vi "工具.vi"() -> ()   [LabVIEW 2011]
panel:
  in  "字符串":string="#0 write #A0 #00 K#00 Z#128@#0 read #A1 #00 #128@#1 write #A0 #00 K#00 Z#128@#1 read #A1 #00 #128$#0 write #A0 #7F V#0@#0 read #A1 #80 #128@#1 write #A0 #7F V#0@#1 read #A1 #80 #128$#0 write #A0 #80 K#01 Z#128@#0 write #A0 #7F V#01@#1 write #A0 #80 K#01 Z#128@#1 write #A0 #7F V#01$#0 write #A0 #7F V#1@#0 read #A1 #80 #128@#1 write #A0 #7F V#1@#1 read #A1 #80 #128$#0 write #A0 #80 K#02 Z#128@#0 write #A0 #7F V#02@#1 write #A0 #80 K#02 Z#128@#1 write #A0 #7F V#02$#0 write #A0 #7F V#2@#0 write #A0 #7B K#10 Z#004@#1 write #A0 #7F V#2@#1 write #A0 #7B K#10 Z#004$#0 write #A0 #7B K#10 Z#004@#0 read #A1 #80 #128@#1 write #A0 #7B K#10 Z#004@#1 read #A1 #80 #128$#0 write #A0 #80 K#03 Z#128@#0 write #A0 #7F V#03@#1 write #A0 #80 K#03 Z#128@#1 write #A0 #7F V#03$#0 write #A0 #7F V#3@#0 read #A1 #80 #128@#1 write #A0 #7F V#3@#1 read #A1 #80 #128$#0 write #A0 #80 K#04 Z#128@#0 write #A0 #7F V#00@#1 write #A0 #80 K#04 Z#128@#1 write #A0 #7F V#00$#0 write #A0 #7F V#0@#0 write #A0 #7B K#11 Z#004@#1 write #A0 #7F V#0@#1 write #A0 #7B K#11 Z#004$#0 write #A0 #7B K#11 Z#004@@#1 write #A0 #7B K#11 Z#004@$@@@$@@@$\r"
  out "电子表格字符串":string="#0 write #A0 #00 K#00 Z#128@#0 read #A1 #00 #128@#1 write #A0 #00 K#00 Z#128@#1 read #A1 #00 #128$#0 write #A0 #7F V#0@#0 read #A1 #80 #128@#1 write #A0 #7F V#0@#1 read #A1 #80 #128$#0 write #A0 #80 K#01 Z#128@#0 write #A0 #7F V#01@#1 write #A0 #80 K#01 Z#128@#1 write #A0 #7F V#01$#0 write #A0 #7F V#1@#0 read #A1 #80 #128@#1 write #A0 #7F V#1@#1 read #A1 #80 #128$#0 write #A0 #80 K#02 Z#128@#0 write #A0 #7F V#02@#1 write #A0 #80 K#02 Z#128@#1 write #A0 #7F V#02$#0 write #A0 #7F V#2@#0 write #A0 #7B K#10 Z#004@#1 write #A0 #7F V#2@#1 write #A0 #7B K#10 Z#004$#0 write #A0 #7B K#10 Z#004@#0 read #A1 #80 #128@#1 write #A0 #7B K#10 Z#004@#1 read #A1 #80 #128$#0 write #A0 #80 K#03 Z#128@#0 write #A0 #7F V#03@#1 write #A0 #80 K#03 Z#128@#1 write #A0 #7F V#03$#0 write #A0 #7F V#3@#0 read #A1 #80 #128@#1 write #A0 #7F V#3@#1 read #A1 #80 #128$#0 write #A0 #80 K#04 Z#128@#0 write #A0 #7F V#00@#1 write #A0 #80 K#04 Z#128@#1 write #A0 #7F V#00$#0 write #A0 #7F V#0@#0 write #A0 #7B K#11 Z#004@#1 write #A0 #7F V#0@#1 write #A0 #7B K#11 Z#004$#0 write #A0 #7B K#11 Z#004@@#1 write #A0 #7B K#11 Z#004@$@@@$@@@$@@@$"
  out "数组":string[][](array[string])=[["#0 write #A0 #00 K#00 Z#128", "#0 read #A1 #00 #128", "#1 write #A0 #00 K#00 Z#128", "#1 read #A1 #00 #128"], ["#0 write #A0 #7F V#0", "#0 read #A1 #80 #128", "#1 write #A0 #7F V#0", "#1 read #A1 #80 #128"], ["#0 write #A0 #80 K#01 Z#128", "#0 write #A0 #7F V#01", "#1 write #A0 #80 K#01 Z#128", "#1 write #A0 #7F V#01"], ["#0 write #A0 #7F V#1", "#0 read #A1 #80 #128", "#1 write #A0 #7F V#1", "#1 read #A1 #80 #128"], ["#0 write #A0 #80 K#02 Z#128", "#0 write #A0 #7F V#02", "#1 write #A0 #80 K#02 Z#128", "#1 write #A0 #7F V#02"], ["#0 write #A0 #7F V#2", "#0 write #A0 #7B K#10 Z#004", "#1 write #A0 #7F V#2", "#1 write #A0 #7B K#10 Z#004"], ["#0 write #A0 #7B K#10 Z#004", "#0 read #A1 #80 #128", "#1 write #A0 #7B K#10 Z#004", "#1 read #A1 #80 #128"], ["#0 write #A0 #80 K#03 Z#128", "#0 write #A0 #7F V#03", "#1 write #A0 #80 K#03 Z#128", "#1 write #A0 #7F V#03"], ["#0 write #A0 #7F V#3", "#0 read #A1 #80 #128", "#1 write #A0 #7F V#3", "#1 read #A1 #80 #128"], ["#0 write #A0 #80 K#04 Z#128", "#0 write #A0 #7F V#00", "#1 write #A0 #80 K#04 Z#128", "#1 write #A0 #7F V#00"], ["#0 write #A0 #7F V#0", "#0 write #A0 #7B K#11 Z#004", "#1 write #A0 #7F V#0", "#1 write #A0 #7B K#11 Z#004"], ["#0 write #A0 #7B K#11 Z#004", "", "#1 write #A0 #7B K#11 Z#004", ""], ["", "", "", ""], ["", "", "", ""], ["", "", "", ""]]
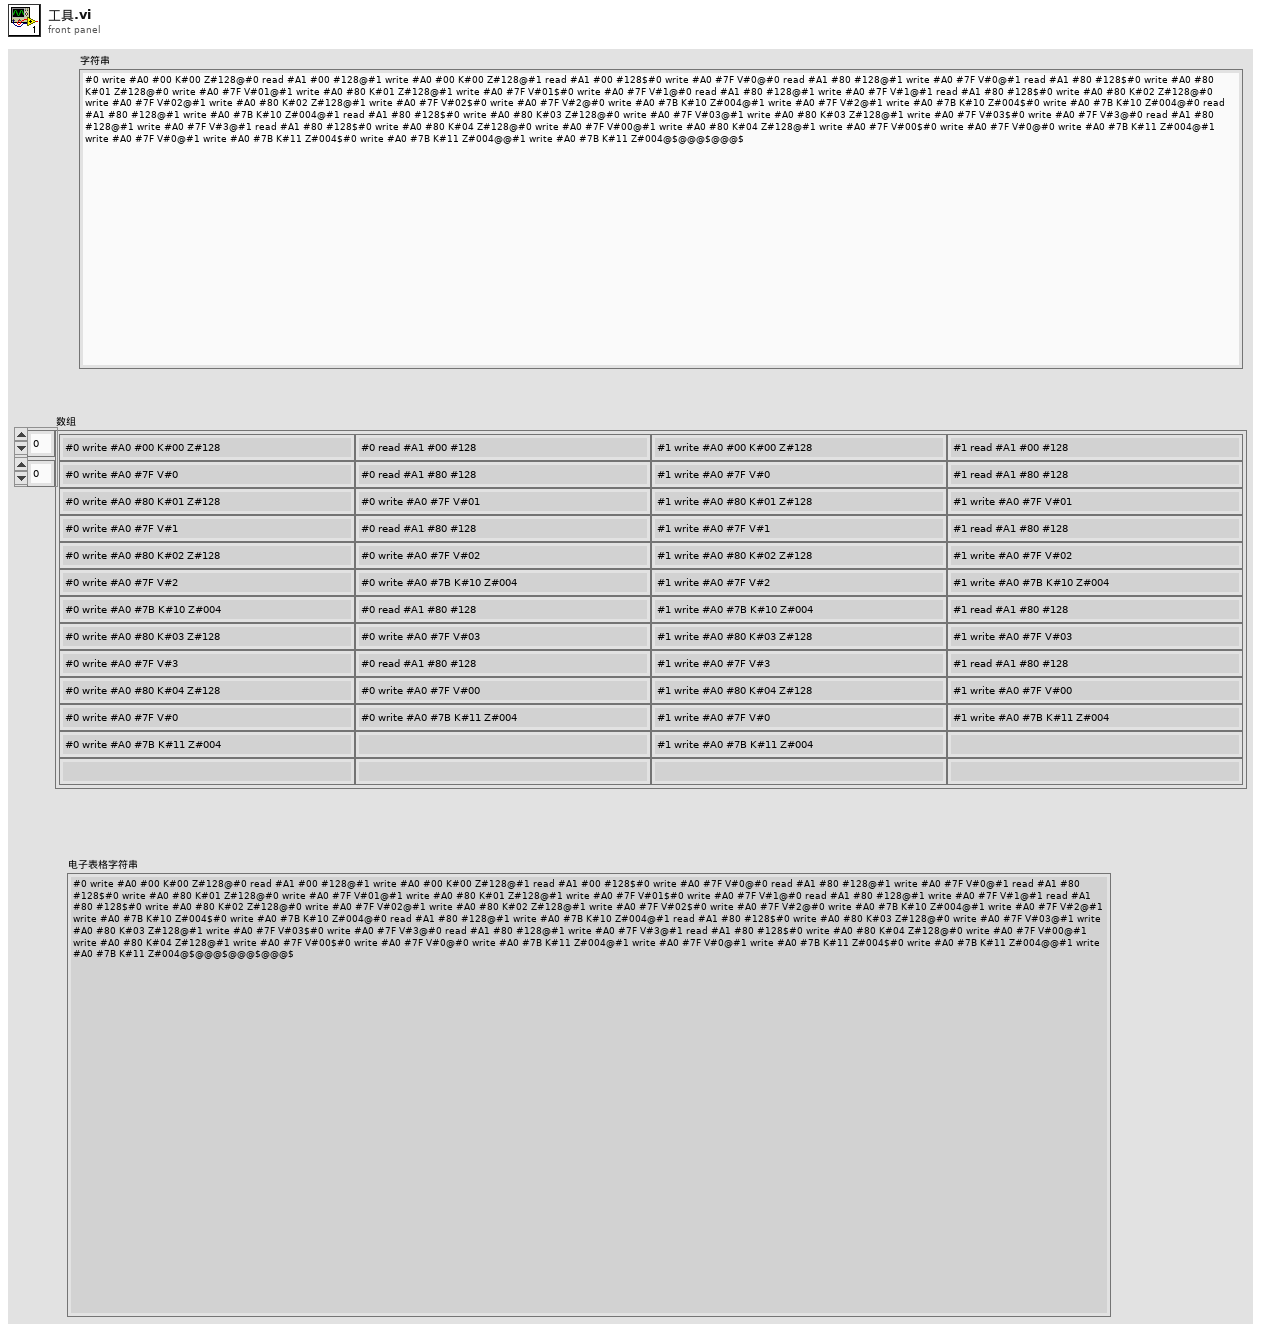
[diagram p1: front panel]
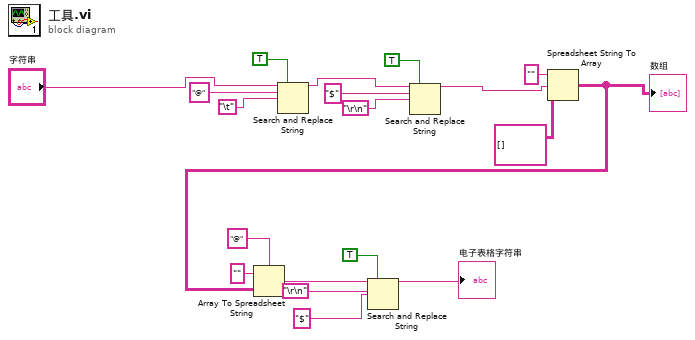
[diagram p0: block diagram]
diagram:
  n1 = Search and Replace String(replace all?=TRUE ("替换全部？(F)"), input string="字符串", search string="@" ("搜索字符串"), replace string="\t") -> (result string=w10:string)  [unwired: 4 in, 3 out]
  n2 = Search and Replace String(replace all?=TRUE ("替换全部？(F)"), input string=w10, search string="$" ("搜索字符串"), replace string="\r\n") -> (result string=w9:string)  [unwired: 4 in, 3 out]
  n3 = Spreadsheet String To Array(format string="" ("格式字符串"), spreadsheet string=w9, array type (2D Dbl)=string[][] []) -> (array=w1:string[][])  [unwired: 1 in]
  "数组" <- w1
  n4 = Array To Spreadsheet String(delimiter (Tab)="@" ("分隔符(Tab)"), array=w1, 3:"" ("格式字符串")) -> (spreadsheet string=w6:string)
  n5 = Search and Replace String(replace all?=TRUE ("替换全部？(F)"), input string=w6, search string="\r\n", replace string="$") -> (result string=→"电子表格字符串":string)  [unwired: 4 in, 3 out]
